vi "getNotificationSettings.vi"(8 "error in (no error)":errorcluster, 11 "reference in":refnum<class "File Controller.lvclass">) -> (0 "error out":errorcluster, 3 "reference out":refnum<class "File Controller.lvclass">)   [LabVIEW 2015, in "File Controller.lvclass"]
uses:
  File Controller.lvclass
  <vilib>/Utility/config.llb/Read Key (Boolean).vi
  <vilib>/Utility/config.llb/NI_LVConfig.lvlib
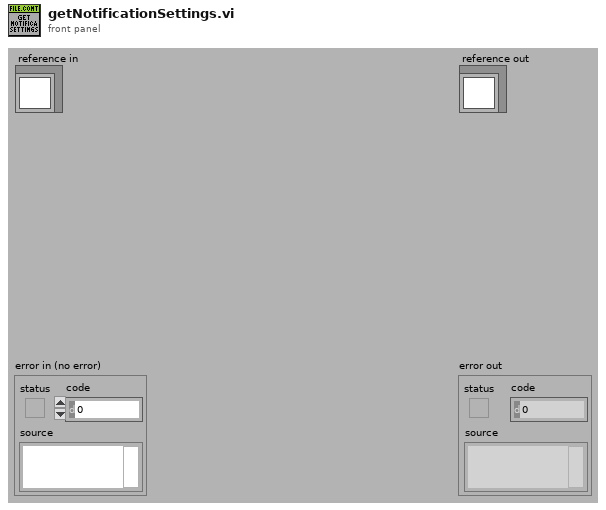
[diagram p1: front panel]
types:
  T1 = typedef "NI_LVConfig.lvlib/Config Data RefNum.ctl" = refnum<k1>
  T2 = typedef "File Controller.lvclass/ObjectAttributesRef.ctl" = refnum<data-value>
  T3 = typedef "File Controller.lvclass/ObjectAttributes.ctl" = cluster{"MyAttribute":dbl, "excelFile_refs":refnum<class "excelFile.lvclass">[], "filePaths":path[], "outlookTemplatePaths":path[], "attachmentTemplatePaths":path[], "configFilePath":path, "not_setting":bool[], "python_ref":refnum<class "python.lvclass">, "TSR":cluster{"number":string, "TSR_path":path, "service_path":path}}
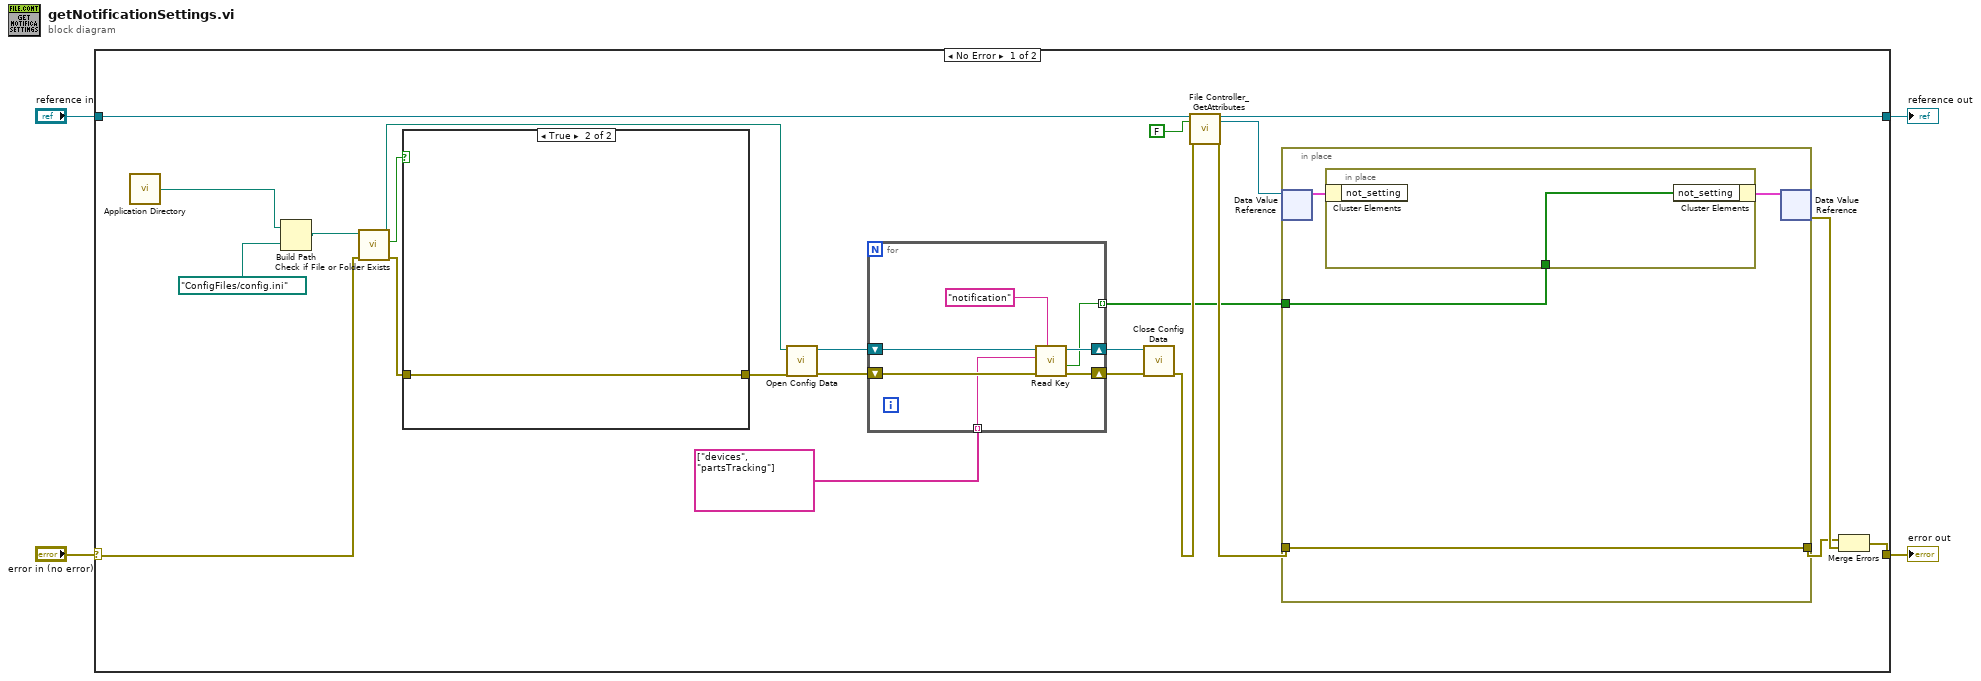
[diagram p0: block diagram]
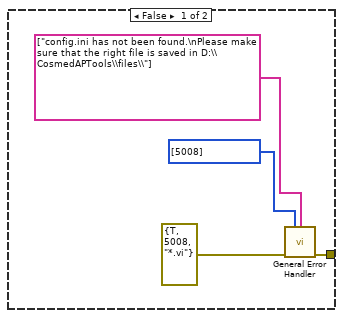
[diagram p2: hidden frame]
diagram:
  n1 = case shown="No Error" "error in (no error)" {
    selector: "error in (no error)" -> [w10 w46]
    tunnel: [w27 w46] -> w3
    tunnel: [w21 w45] -> w1
    tunnel: "reference in" -> [w24 w45]
    frame No Error {
      n2 = call <vilib>:"Application Directory.vi"() -> ("Application Directory"=w6:path)
      n3 = Build Path(base path=w6, name or relative path=path "ConfigFiles/config.ini" ("path")) -> (appended path=w5:path)
      n4 = call <vilib>:"Check if File or Folder Exists.vi"("error in (no error)"=w10, "path"=w5) -> ("error out"=w19:errorcluster, "file or folder exists?"=w18:bool, "dup path"=w16:path)  [unwired: 7 in]
      n5 = case shown="True" w18 {
        tunnel: w19 -> [_ w39]
        tunnel: [w38 w39] -> w17
        frame False {
          n6 = call <vilib>:"General Error Handler.vi"("[user-defined codes]"=i32[] [5008], "[user-defined descriptions]"=string[] ["config.ini has not been found.\nPlease make sure that the right file is saved in D:\\CosmedAPTools\\files\\"], "error in (no error)"=errorcluster {"status"=TRUE, "code"=5008, "source"="*.vi"}) -> ("error out"=w38:errorcluster)  [unwired: 8 in, 4 out]
        }
        frame True {
        }
      }
      n7 = call <vilib>:"Open Config Data.vi"("error in (no error)"=w17, "configuration file path"=w16) -> ("error out"=w14:errorcluster, "refnum"=w15:T1)  [unwired: 7 in, 1 out]
      n8 = for {
        shift-right: [w31] -> w13
        shift-left: w15 -> [w34]
        shift-right: [w30] -> w12
        shift-left: w14 -> [w33]
        tunnel: string[] ["devices", "partsTracking"] -> [w29] mode=indexing
        tunnel: [w28] -> w8 mode=indexing
        n9 = call-poly <vilib>:"Read Key.vi"("section"="notification", "error in (no error)"=w33, "key"=w29, "refnum"=w34) -> ("error out"=w30:errorcluster, "value"=w28:bool, "refnum out"=w31:T1)  [unwired: 4 in, 1 out]
      }
      n10 = call <vilib>:"Close Config Data.vi"("error in (no error)"=w12, "refnum"=w13) -> ("error out"=w9:errorcluster)  [unwired: 8 in, 1 out]
      n11 = call "File Controller_GetAttributes.vi"("reference in"=w24, "return data? (T)"=FALSE, "error in (no error)"=w9) -> ("reference out"=w21:refnum<class "File Controller.lvclass">, "attributes ref"=w20:T2, "error out"=w22:errorcluster)  [unwired: 13 in, 1 out]
      n12 = in-place {
        in-place-border: w22 -> [w41]
        in-place-border: [w41] -> w25
        in-place-border: w8 -> [w40]
        n13 = in-place-dvr #1(w20) -> (w42:T3)  [unwired: 1 out]
        n14 = in-place {
          in-place-border: w40 -> [w44]
          n15 = in-place-cluster #2(w42) -> ()  [unwired: 1 out]
          n16 = in-place-cluster #2("not_setting"=w44) -> (w43:T3)
        }
        n17 = in-place-dvr #1(w43) -> (w26:errorcluster)  [unwired: 1 out]
      }
      n18 = Merge Errors(w25, w26) -> (w27:errorcluster)
    }
    frame Error {
    }
  }
  "error out" <- w3
  "reference out" <- w1
